vi "SetModeSettings.vi"(8 "error in (no error)":errorcluster, 10 "Mode":T1, 11 "Drive.lvlib:Pod Drive.lvclass":refnum<class "Pod Drive.lvclass">) -> (0 "error out":errorcluster, 3 "?":refnum<class "Pod Drive.lvclass">)   [LabVIEW 2018, in "Drive.lvlib" / "Pod Drive.lvclass"]
doc: "This VI sets constants on the drive train for different modes of operation."
uses:
  Pod Drive.lvclass
  Controls/Mode.ctl
  C:/Users/Public/Documents/2019DeepSpace/Classes/Drive/Drive.lvclass
  Pod Drive.lvclass/Pod Drive.ctl
  <vilib>/Rock Robotics/WPI/ThirdParty/Phoenix-LabVIEW/Motor Controller/Controls/CTRE_Phoenix_MotorControl_EnhancedMotorControllerConfigurables.ctl
  <vilib>/Rock Robotics/WPI/ThirdParty/Phoenix-LabVIEW/Motor Controller/Controls/CTRE_Phoenix_MotorControl_BaseConfigurables.ctl
  <vilib>/Rock Robotics/WPI/ThirdParty/Phoenix-LabVIEW/Motor Controller/Controls/CTRE_Phoenix_MotorControl_VelocityMeasurementPeriod.ctl
  <vilib>/Rock Robotics/WPI/ThirdParty/Phoenix-LabVIEW/Motor Controller/Controls/CTRE_Phoenix_MotorControl_SlotStructure.ctl
  <vilib>/Rock Robotics/WPI/ThirdParty/Phoenix-LabVIEW/Motor Controller/Controls/CTRE_Phoenix_MotorControl_FilterStruct.ctl
  <vilib>/Rock Robotics/WPI/ThirdParty/Phoenix-LabVIEW/Motor Controller/Controls/CTRE_Phoenix_MotorControl_RemoteSourceType.ctl
  <vilib>/Rock Robotics/WPI/ThirdParty/Phoenix-LabVIEW/Controls/CTRE_Phoenix_CustomParamConfiguration.ctl
  <vilib>/Rock Robotics/WPI/ThirdParty/Phoenix-LabVIEW/Motor Controller/Controls/CTRE_Phoenix_MotorControl_FeedbackDevice.ctl
  <vilib>/Rock Robotics/WPI/ThirdParty/Phoenix-LabVIEW/Motor Controller/Controls/CTRE_Phoenix_MotorControl_SensorTermFeedbackDevice_Enhanced.ctl
  <vilib>/Rock Robotics/WPI/ThirdParty/Phoenix-LabVIEW/Motor Controller/Controls/CTRE_Phoenix_MotorControl_LimitSwitchNormal.ctl
  <vilib>/Rock Robotics/WPI/ThirdParty/Phoenix-LabVIEW/Motor Controller/Controls/CTRE_Phoenix_MotorControl_LimitSwitchSource_Local.ctl
  Drive.lvclass/Drive.ctl
  Public Methods/Read Drive Motion Magic Primary Low Gear.vi
  Public Methods/Read Drive Motion Magic Primary High Gear.vi
  Public Methods/Read Drive Motion Magic Secondary Low Gear.vi
  Public Methods/Read Drive Motion Magic Secondary High Gear.vi
  Public Methods/Read Motion Magic Constants.vi
  Public Methods/Read Drive Velocity Low Gear.vi
  Public Methods/Read Drive Velocity High Gear.vi
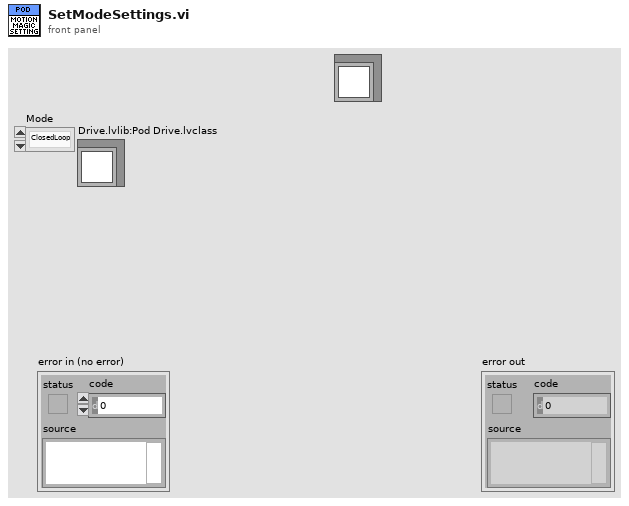
[diagram p1: front panel]
types:
  T1 = typedef "Drive.lvlib/Pod Drive.lvclass/Mode.ctl" = enum16{"ClosedLoop", "MotionMagic"}
  T2 = typedef "CTRE_Phoenix_MotorControl_EnhancedMotorControllerConfigurables.ctl" = cluster{"Base Configurables":T3, "primaryPID":cluster{"selectedFeedbackCoefficient":dbl, "selectedFeedbackSensor":T9}, "auxiliaryPID":cluster{"selectedFeedbackCoefficient":dbl, "selectedFeedbackSensor":T9}, "sum0Term":T10, "sum1Term":T10, "diff0Term":T10, "diff1Term":T10, "forwardLimitSwitchNormal":T11, "reverseLimitSwitchNormal":T11, "forwardLimitSwitchDeviceID":i32, "reverseLimitSwitchDeviceID":i32, "forwardLimitSwitchSource":T12, "reverseLimitSwitchSource":T12, "peakCurrentLimit":i32, "peakCurrentDuration":i32, "continuousCurrentLimit":i32}
  T3 = typedef "CTRE_Phoenix_MotorControl_BaseConfigurables.ctl" = cluster{"openLoopRamp":dbl, "closedLoopRamp":dbl, "peakOutputForward":dbl, "peakOutputReverse":dbl, "nominalOutputForward":dbl, "nominalOutputReverse":dbl, "neutralDeadband":dbl, "voltageCompSaturation":dbl, "voltageMeasurementFilter":i32, "velocityMeasurementPeriod":T4, "velocityMeasurementWindow":i32, "forwardSoftLimitThreshold":i32, "reverseSoftLimitThreshold":i32, "forwardSoftLimitEnable":bool, "reverseSoftLimitEnable":bool, "slot0":T5, "slot1":T5, "slot2":T5, "slot3":T5, "auxPIDPolarity":bool, "remoteFilter0":T6, "remoteFilter1":T6, "motionCruiseVelocity":i32, "motionAcceleration":i32, "motionProfileTrajectoryPeriod":i32, "feedbackNotContinuous":bool, "remoteSensorClosedLoopDisableNeutralOnLOS":bool, "clearPositionOnLimitF":bool, "clearPositionOnLimitR":bool, "clearPositionOnQuadIdx":bool, "limitSwitchDisableNeutralOnLOS":bool, "softLimitDisableNeutralOnLOS":bool, "pulseWidthPeriod_EdgesPerRot":i32, "pulseWidthPeriod_FilterWindowSz":i32, "customParam":T8, "trajectoryInterpolationEnable":bool}
  T4 = typedef "CTRE_Phoenix_MotorControl_VelocityMeasurementPeriod.ctl" = u16
  T5 = typedef "CTRE_Phoenix_MotorControl_SlotStructure.ctl" = cluster{"P":dbl, "I":dbl, "D":dbl, "F":dbl, "integralZone":dbl, "allowableClosedLoopError":i32, "maxIntegralAccumulator":dbl, "closedLoopPeakOutput":dbl, "closedLoopPeriod":i32}
  T6 = typedef "CTRE_Phoenix_MotorControl_FilterStruct.ctl" = cluster{"remoteSensorDeviceID":u8, "remoteSensorSource":T7}
  T7 = typedef "CTRE_Phoenix_MotorControl_RemoteSourceType.ctl" = enum16{"Off", "Talon SRX Selected Sensor", "Pigeon IMU Yaw", "Pigeon IMU Pitch", "Pigeon IMU Roll", "CANifier Quadrature", "CANifier PWM Input 0", "CANifier PWM Input 1", "CANifier PWM Input 2", "CANifier PWM Input 3", "Gadgeteer Pigeon Yaw", "Gadgeteer Pigeon Pitch", "Gadgeteer Pigeon Roll"}
  T8 = typedef "CTRE_Phoenix_CustomParamConfiguration.ctl" = cluster{"customParam0":i32, "customParam1":i32}
  T9 = typedef "CTRE_Phoenix_MotorControl_FeedbackDevice.ctl" = i8
  T10 = typedef "CTRE_Phoenix_MotorControl_SensorTermFeedbackDevice_Enhanced.ctl" = i8
  T11 = typedef "CTRE_Phoenix_MotorControl_LimitSwitchNormal.ctl" = enum16{"Normally Open", "Normally Closed", "Disabled"}
  T12 = typedef "CTRE_Phoenix_MotorControl_LimitSwitchSource_Local.ctl" = enum16{"Feedback Connector", "Remote Talon SRX", "Remote CANifier", "Deactivated"}
  T13 = enum16{"FollowerType_PercentOutput", "FollowerType_AuxOutput1"}
  T14 = typedef "Drive.lvlib/Drive.lvclass/Motion Magic Constants.ctl" = cluster{"Low Gear Max Velocity":u32, "High Gear Max Velocity":u32, "Motion Magic Low Gear Max Velocity":u32, "Motion Magic Low Gear Max Acceleration":u32, "Motion Magic High Gear Max Velocity":u32, "Motion Magic High Gear Max Acceleration":u32}
  T15 = typedef "WPI_MotorControlDeviceRef.ctl" = cluster{"DeviceStatus":errorcluster, "Type":T16, "PWM":cluster{"PWM Channel":T17, "DeadBand":T18}, "CAN":cluster{"Device Number":u8, "SetOutput VI Ref":variant, "GetOutput VI Ref":variant, "Enable VI Ref":variant, "Disable VI Ref":variant, "Data":variant}, "Invert":bool, "DIO PWM":cluster{"PWM \"Enable\" Channel":T17, "DIOChannel":T19, "PWM Rate":dbl}}
  T16 = typedef "WPI_MotorControlType.ctl" = enum16{"PWM", "CAN", "DIO PWM"}
  T17 = typedef "FPGA_DIOPWMChannel.ctl" = enum8{"PWM 0", "PWM 1", "PWM 2", "PWM 3", "PWM 4", "PWM 5", "PWM 6", "PWM 7", "PWM 8", "PWM 9", "PWM MXP 0", "PWM MXP 1", "PWM MXP 2", "PWM MXP 3", "PWM MXP 4", "PWM MXP 5", "PWM MXP 6", "PWM MXP 7", "PWM MXP 8", "PWM MXP 9", "Invalid"}
  T18 = typedef "WPI_PWMDeadband.ctl" = cluster{"Name":string, "maxPositivePwm":i32, "minPositivePwm":i32, "centerPwm":i32, "maxNegativePwm":i32, "minNegativePwm":i32, "angularRange":u16}
  T19 = typedef "FPGA_DIOChannel.ctl" = enum8{"DIO 0", "DIO 1", "DIO 2", "DIO 3", "DIO 4", "DIO 5", "DIO 6", "DIO 7", "DIO 8", "DIO 9", "DIO MXP 0", "DIO MXP 1", "DIO MXP 2", "DIO MXP 3", "DIO MXP 4", "DIO MXP 5", "DIO MXP 6", "DIO MXP 7", "DIO MXP 8", "DIO MXP 9", "DIO MXP 10", "DIO MXP 11", "DIO MXP 12", "DIO MXP 13", "DIO MXP 14", "DIO MXP 15", "SPI Port CS1", "SPI Port CS2", "SPI Port CS3", "SPI Port MISO", "SPI Port MOSI", "Invalid"}
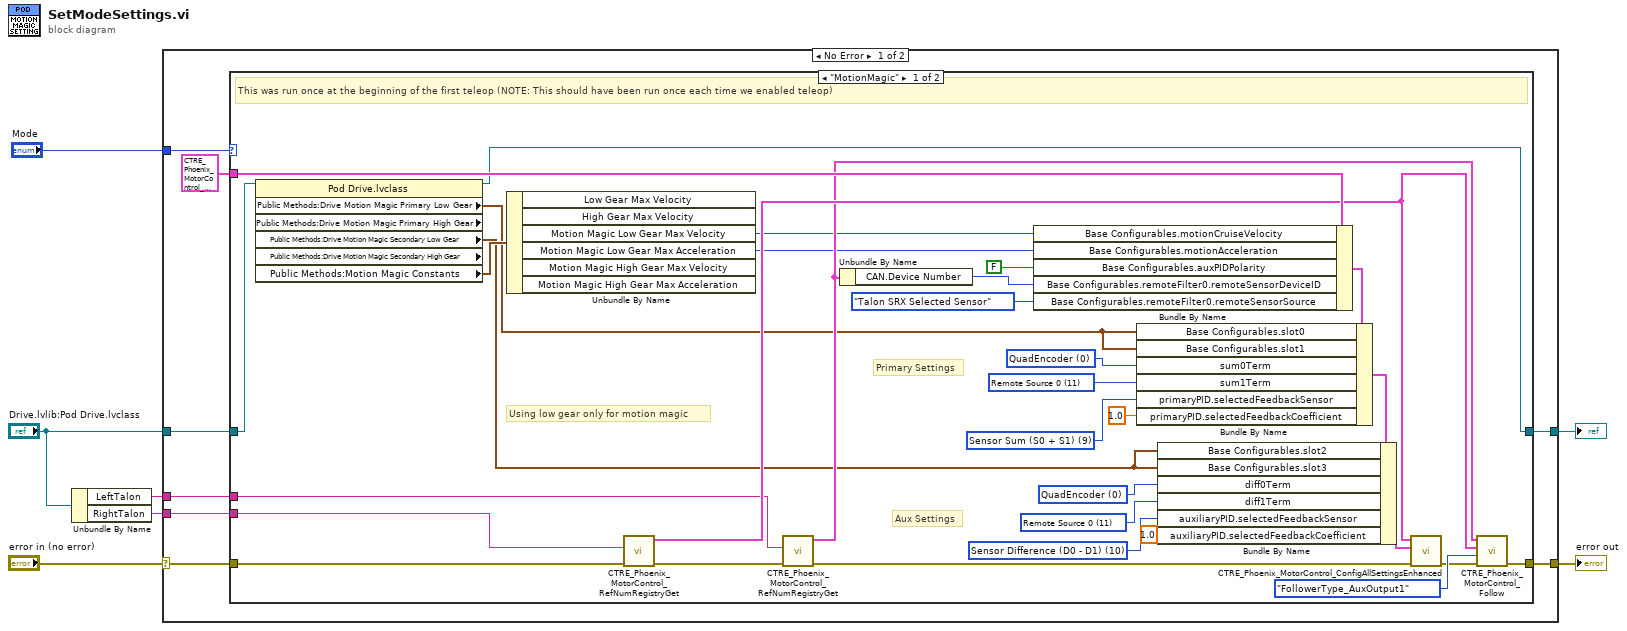
[diagram p0: block diagram]
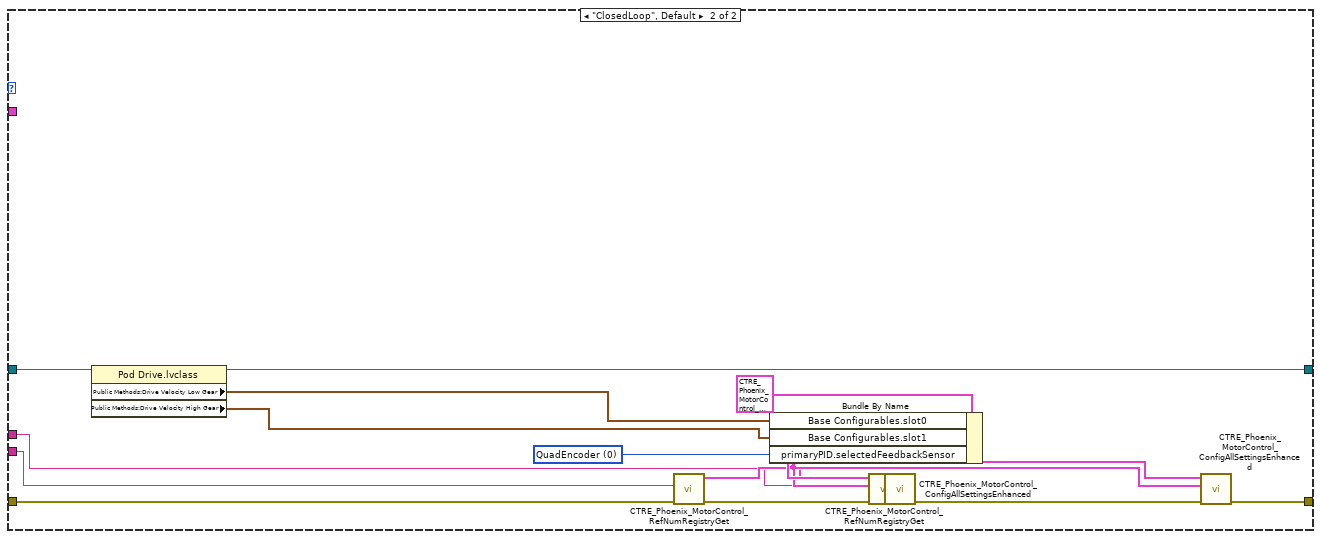
[diagram p2: hidden frame]
diagram:
  n1 = Unbundle By Name("Drive.lvlib:Pod Drive.lvclass") -> ("LeftTalon"=w4:string, "RightTalon"=w3:string)
  n2 = case shown="No Error" "error in (no error)" {
    selector: "error in (no error)" -> [w15 w65]
    tunnel: [w14 w65] -> w6
    tunnel: "Mode" -> [w13 _]
    tunnel: w3 -> [w11 _]
    tunnel: w4 -> [w10 _]
    tunnel: "Drive.lvlib:Pod Drive.lvclass" -> [w9 w64]
    tunnel: [w8 w64] -> w1
    frame No Error {
      n3 = case shown="\"MotionMagic\"" w13 {
        tunnel: [w44 w58] -> w14
        tunnel: w15 -> [w40 w57]
        tunnel: T2 {"Base Configurables"={"openLoopRamp"=0.0, "closedLoopRamp"=0.0, "peakOutputForward"=1.0, "peakOutputReverse"=-1.0, "nominalOutputForward"=0.0, "nominalOutputReverse"=0.0, "neutralDeadband"=0.04, "voltageCompSaturation"=0.0, "voltageMeasurementFilter"=32, "velocityMeasurementPeriod"=100, "velocityMeasurementWindow"=64, "forwardSoftLimitThreshold"=0, "reverseSoftLimitThreshold"=0, "forwardSoftLimitEnable"=FALSE, "reverseSoftLimitEnable"=FALSE, "slot0"={"P"=0.0, "I"=0.0, "D"=0.0, "F"=0.0, "integralZone"=0.0, "allowableClosedLoopError"=0, "maxIntegralAccumulator"=0.0, "closedLoopPeakOutput"=1.0, "closedLoopPeriod"=1}, "slot1"={"P"=0.0, "I"=0.0, "D"=0.0, "F"=0.0, "integralZone"=0.0, "allowableClosedLoopError"=0, "maxIntegralAccumulator"=0.0, "closedLoopPeakOutput"=1.0, "closedLoopPeriod"=1}, "slot2"={"P"=0.0, "I"=0.0, "D"=0.0, "F"=0.0, "integralZone"=0.0, "allowableClosedLoopError"=0, "maxIntegralAccumulator"=0.0, "closedLoopPeakOutput"=1.0, "closedLoopPeriod"=1}, "slot3"={"P"=0.0, "I"=0.0, "D"=0.0, "F"=0.0, "integralZone"=0.0, "allowableClosedLoopError"=0, "maxIntegralAccumulator"=0.0, "closedLoopPeakOutput"=1.0, "closedLoopPeriod"=1}, "auxPIDPolarity"=FALSE, "remoteFilter0"={"remoteSensorDeviceID"=0, "remoteSensorSource"=enum."Off"}, "remoteFilter1"={"remoteSensorDeviceID"=0, "remoteSensorSource"=enum."Off"}, "motionCruiseVelocity"=0, "motionAcceleration"=0, "motionProfileTrajectoryPeriod"=0, "feedbackNotContinuous"=FALSE, "remoteSensorClosedLoopDisableNeutralOnLOS"=FALSE, "clearPositionOnLimitF"=FALSE, "clearPositionOnLimitR"=FALSE, "clearPositionOnQuadIdx"=FALSE, "limitSwitchDisableNeutralOnLOS"=FALSE, "softLimitDisableNeutralOnLOS"=FALSE, "pulseWidthPeriod_EdgesPerRot"=1, "pulseWidthPeriod_FilterWindowSz"=1, "customParam"={"customParam0"=0, "customParam1"=0}, "trajectoryInterpolationEnable"=TRUE}, "primaryPID"={"selectedFeedbackCoefficient"=1.0, "selectedFeedbackSensor"=0}, "auxiliaryPID"={"selectedFeedbackCoefficient"=1.0, "selectedFeedbackSensor"=0}, "sum0Term"=0, "sum1Term"=0, "diff0Term"=0, "diff1Term"=0, "forwardLimitSwitchNormal"=enum."Normally Open", "reverseLimitSwitchNormal"=enum."Normally Open", "forwardLimitSwitchDeviceID"=0, "reverseLimitSwitchDeviceID"=0, "forwardLimitSwitchSource"=enum."Feedback Connector", "reverseLimitSwitchSource"=enum."Feedback Connector", "peakCurrentLimit"=1, "peakCurrentDuration"=1, "continuousCurrentLimit"=1} ("Enhanced Motor Controller Configurables") -> [w37 _]
        tunnel: w11 -> [w24 w54]
        tunnel: w10 -> [w23 w55]
        tunnel: w9 -> [w22 w51]
        tunnel: [w16 w50] -> w8
        frame "MotionMagic" {
          w27 = T9 10 items=["QuadEncoder"=0, "Analog"=2, "Tachometer"=4, "Pulse Width Encoded Position"=8, "Sensor Sum (S0 + S1)"=9, "Sensor Difference (D0 - D1)"=10, "Remote Source 0"=11, "Remote Source 1"=12, "Software Emulated"=15] ("auxiliaryPID.selectedFeedbackSensor")
          w28 = T10 11 items=["QuadEncoder"=0, "Analog"=2, "Tachometer"=4, "Pulse Width Encoded Position"=8, "Remote Source 0"=11, "Remote Source 1"=12, "Software Emulated"=15] ("diff1Term")
          w29 = T10 0 items=["QuadEncoder"=0, "Analog"=2, "Tachometer"=4, "Pulse Width Encoded Position"=8, "Remote Source 0"=11, "Remote Source 1"=12, "Software Emulated"=15] ("diff0Term")
          w31 = T9 9 items=["QuadEncoder"=0, "Analog"=2, "Tachometer"=4, "Pulse Width Encoded Position"=8, "Sensor Sum (S0 + S1)"=9, "Sensor Difference (D0 - D1)"=10, "Remote Source 0"=11, "Remote Source 1"=12, "Software Emulated"=15] ("primaryPID.selectedFeedbackSensor")
          w45 = T10 11 items=["QuadEncoder"=0, "Analog"=2, "Tachometer"=4, "Pulse Width Encoded Position"=8, "Remote Source 0"=11, "Remote Source 1"=12, "Software Emulated"=15] ("sum1Term")
          w46 = T10 0 items=["QuadEncoder"=0, "Analog"=2, "Tachometer"=4, "Pulse Width Encoded Position"=8, "Remote Source 0"=11, "Remote Source 1"=12, "Software Emulated"=15] ("sum0Term")
          # "Using low gear only for motion magic"
          # "Aux Settings"
          # "Primary Settings"
          # "This was run once at the beginning of the first teleop (NOTE: This should have been run once each time we enabled teleop)"
          n4 = property class="Pod Drive.lvclass" props=["Public Methods:Drive Motion Magic Primary Low Gear", "Public Methods:Drive Motion Magic Primary High Gear", "Public Methods:Drive Motion Magic Secondary Low Gear", "Public Methods:Drive Motion Magic Secondary High Gear", "Public Methods:Motion Magic Constants"](reference=w22) -> (reference out=w16:refnum<class "Pod Drive.lvclass">, "Public Methods:Drive Motion Magic Primary Low Gear"=w19:T5, "Public Methods:Drive Motion Magic Secondary Low Gear"=w20:T5, "Public Methods:Motion Magic Constants"=w21:T14)  [unwired: 1 in, 3 out]
          n5 = Unbundle By Name(w21) -> ("Motion Magic Low Gear Max Velocity"=w18:u32, "Motion Magic Low Gear Max Acceleration"=w17:u32)  [unwired: 4 out]
          n6 = call <vilib>:"CTRE_Phoenix_MotorControl_RefNumRegistryGet.vi"("error in (no error)"=w40, "refnum name"=w24) -> ("error out"=w41:errorcluster, "PhoenixMotorControlDevRef"=w34:T15)  [unwired: 8 in]
          n7 = call <vilib>:"CTRE_Phoenix_MotorControl_RefNumRegistryGet.vi"("error in (no error)"=w41, "refnum name"=w23) -> ("error out"=w42:errorcluster, "PhoenixMotorControlDevRef"=w25:T15)  [unwired: 8 in]
          n8 = Unbundle By Name(w25) -> ("CAN.Device Number"=w33:u8)
          n9 = Bundle By Name(cluster=w37, "Base Configurables.motionCruiseVelocity"=w18, "Base Configurables.motionAcceleration"=w17, "Base Configurables.auxPIDPolarity"=FALSE, "Base Configurables.remoteFilter0.remoteSensorDeviceID"=w33, "Base Configurables.remoteFilter0.remoteSensorSource"=CTRE_Phoenix_MotorControl_RemoteSourceType."Talon SRX Selected Sensor") -> (w36:T2)
          n10 = Bundle By Name(cluster=w36, "Base Configurables.slot0"=w19, "Base Configurables.slot1"=w19, "sum0Term"=w46, "sum1Term"=w45, "primaryPID.selectedFeedbackSensor"=w31, "primaryPID.selectedFeedbackCoefficient"=1.0) -> (w39:T2)
          n11 = Bundle By Name(cluster=w39, "Base Configurables.slot2"=w20, "Base Configurables.slot3"=w20, "diff0Term"=w29, "diff1Term"=w28, "auxiliaryPID.selectedFeedbackSensor"=w27, "auxiliaryPID.selectedFeedbackCoefficient"=1.0) -> (w38:T2)
          n12 = call <vilib>:"CTRE_Phoenix_MotorControl_ConfigAllSettingsEnhanced.vi"("error in (no error)"=w42, "Enhanced Motor Controller Configurables"=w38, "PhoenixMotorControlDevRef"=w34) -> ("error out"=w43:errorcluster)  [unwired: 7 in, 1 out]
          n13 = call <vilib>:"CTRE_Phoenix_MotorControl_Follow.vi"("error in (no error)"=w43, "FollowerType"=T13."FollowerType_AuxOutput1", "Master Controller to Follow"=w34, "PhoenixMotorControlDevRef"=w25) -> ("error out"=w44:errorcluster)  [unwired: 6 in, 1 out]
        }
        frame "ClosedLoop", Default {
          w56 = T9 0 items=["QuadEncoder"=0, "Analog"=2, "Tachometer"=4, "Pulse Width Encoded Position"=8, "Sensor Sum (S0 + S1)"=9, "Sensor Difference (D0 - D1)"=10, "Remote Source 0"=11, "Remote Source 1"=12, "Software Emulated"=15] ("primaryPID.selectedFeedbackSensor")
          n14 = property class="Pod Drive.lvclass"(reference=w51) -> (reference out=w50:refnum<class "Pod Drive.lvclass">, "Public Methods:Drive Velocity Low Gear"=w49:T5, "Public Methods:Drive Velocity High Gear"=w48:T5)  [unwired: 1 in, 1 out]
          n15 = call <vilib>:"CTRE_Phoenix_MotorControl_RefNumRegistryGet.vi"("error in (no error)"=w57, "refnum name"=w54) -> ("error out"=w53:errorcluster, "PhoenixMotorControlDevRef"=w60:T15)  [unwired: 8 in]
          n16 = Bundle By Name(cluster=T2 {"Base Configurables"={"openLoopRamp"=0.0, "closedLoopRamp"=0.0, "peakOutputForward"=1.0, "peakOutputReverse"=-1.0, "nominalOutputForward"=0.0, "nominalOutputReverse"=0.0, "neutralDeadband"=0.04, "voltageCompSaturation"=0.0, "voltageMeasurementFilter"=32, "velocityMeasurementPeriod"=100, "velocityMeasurementWindow"=64, "forwardSoftLimitThreshold"=0, "reverseSoftLimitThreshold"=0, "forwardSoftLimitEnable"=FALSE, "reverseSoftLimitEnable"=FALSE, "slot0"={"P"=0.0, "I"=0.0, "D"=0.0, "F"=0.0, "integralZone"=0.0, "allowableClosedLoopError"=0, "maxIntegralAccumulator"=0.0, "closedLoopPeakOutput"=1.0, "closedLoopPeriod"=1}, "slot1"={"P"=0.0, "I"=0.0, "D"=0.0, "F"=0.0, "integralZone"=0.0, "allowableClosedLoopError"=0, "maxIntegralAccumulator"=0.0, "closedLoopPeakOutput"=1.0, "closedLoopPeriod"=1}, "slot2"={"P"=0.0, "I"=0.0, "D"=0.0, "F"=0.0, "integralZone"=0.0, "allowableClosedLoopError"=0, "maxIntegralAccumulator"=0.0, "closedLoopPeakOutput"=1.0, "closedLoopPeriod"=1}, "slot3"={"P"=0.0, "I"=0.0, "D"=0.0, "F"=0.0, "integralZone"=0.0, "allowableClosedLoopError"=0, "maxIntegralAccumulator"=0.0, "closedLoopPeakOutput"=1.0, "closedLoopPeriod"=1}, "auxPIDPolarity"=FALSE, "remoteFilter0"={"remoteSensorDeviceID"=0, "remoteSensorSource"=enum."Off"}, "remoteFilter1"={"remoteSensorDeviceID"=0, "remoteSensorSource"=enum."Off"}, "motionCruiseVelocity"=0, "motionAcceleration"=0, "motionProfileTrajectoryPeriod"=0, "feedbackNotContinuous"=FALSE, "remoteSensorClosedLoopDisableNeutralOnLOS"=FALSE, "clearPositionOnLimitF"=FALSE, "clearPositionOnLimitR"=FALSE, "clearPositionOnQuadIdx"=FALSE, "limitSwitchDisableNeutralOnLOS"=FALSE, "softLimitDisableNeutralOnLOS"=FALSE, "pulseWidthPeriod_EdgesPerRot"=1, "pulseWidthPeriod_FilterWindowSz"=1, "customParam"={"customParam0"=0, "customParam1"=0}, "trajectoryInterpolationEnable"=TRUE}, "primaryPID"={"selectedFeedbackCoefficient"=1.0, "selectedFeedbackSensor"=0}, "auxiliaryPID"={"selectedFeedbackCoefficient"=1.0, "selectedFeedbackSensor"=0}, "sum0Term"=0, "sum1Term"=0, "diff0Term"=0, "diff1Term"=0, "forwardLimitSwitchNormal"=enum."Normally Open", "reverseLimitSwitchNormal"=enum."Normally Open", "forwardLimitSwitchDeviceID"=0, "reverseLimitSwitchDeviceID"=0, "forwardLimitSwitchSource"=enum."Feedback Connector", "reverseLimitSwitchSource"=enum."Feedback Connector", "peakCurrentLimit"=1, "peakCurrentDuration"=1, "continuousCurrentLimit"=1} ("Enhanced Motor Controller Configurables"), "Base Configurables.slot0"=w49, "Base Configurables.slot1"=w48, "primaryPID.selectedFeedbackSensor"=w56) -> (w61:T2)
          n17 = call <vilib>:"CTRE_Phoenix_MotorControl_RefNumRegistryGet.vi"("error in (no error)"=w53, "refnum name"=w55) -> ("error out"=w52:errorcluster, "PhoenixMotorControlDevRef"=w62:T15)  [unwired: 8 in]
          n18 = call <vilib>:"CTRE_Phoenix_MotorControl_ConfigAllSettingsEnhanced.vi"("error in (no error)"=w52, "Enhanced Motor Controller Configurables"=w61, "PhoenixMotorControlDevRef"=w60) -> ("error out"=w59:errorcluster)  [unwired: 7 in, 1 out]
          n19 = call <vilib>:"CTRE_Phoenix_MotorControl_ConfigAllSettingsEnhanced.vi"("error in (no error)"=w59, "Enhanced Motor Controller Configurables"=w61, "PhoenixMotorControlDevRef"=w62) -> ("error out"=w58:errorcluster)  [unwired: 7 in, 1 out]
        }
      }
    }
    frame Error {
    }
  }
  "error out" <- w6
  "?" <- w1
